vi "VI Server_TextRing_Update_ItemNames.vi"(7 "Label":string, 8 "error in":errorcluster, 10 "Strings []":string[](array[string]), 11 "VI Server Cluster":T1) -> (0 "error out":errorcluster, 1 "Control Reference":refnum<vi>, 3 "VI Server Cluster.DUP":T1)   [LabVIEW 2020, in "VI Server Toolkit LV2013.lvlib"]
doc: "Updates Text Ring Items List."
uses:
  VI Server Toolkit LV2013.lvlib
  VI Server_TypeDefs/VI Server_RefsCluster.ctl
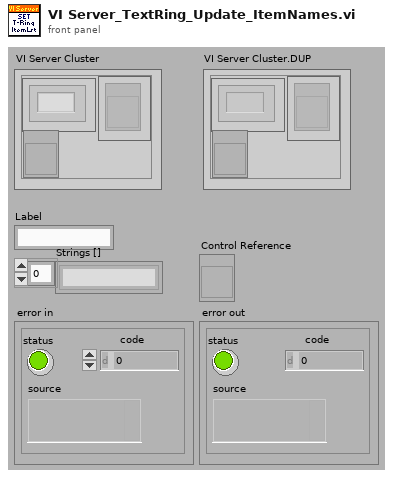
[diagram p1: front panel]
types:
  T1 = typedef "VI Server_RefsCluster.ctl" = cluster{"Labels":string[], "Refs":refnum<vi>[], "VI Ref":refnum<vi>}
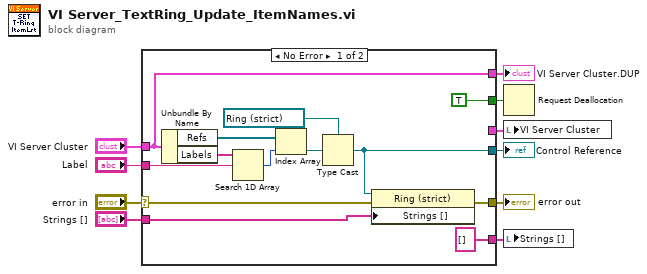
[diagram p0: block diagram]
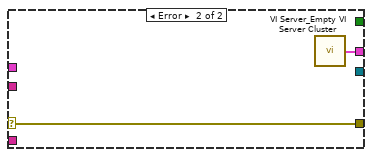
[diagram p2: hidden frame]
diagram:
  n1 = case shown="No Error" "error in" {
    selector: "error in" -> [w17 w25]
    tunnel: "Label" -> [w22 _]
    tunnel: "VI Server Cluster" -> [w13 _]
    tunnel: [w16 w25] -> w10
    tunnel: [w15 _] -> w6
    tunnel: "Strings []" -> [w14 _]
    tunnel: [w13 _] -> w4
    tunnel: [_ w24] -> w3
    tunnel: [string[] [] ("Strings []") _] -> w2
    tunnel: [TRUE _] -> w1
    frame No Error {
      n2 = Unbundle By Name(w13) -> ("Refs"=w20:refnum<vi>[], "Labels"=w23:string[])
      n3 = Search 1D Array(1D array=w23, element=w22) -> (index of element=w21:i32)  [unwired: 1 out]
      n4 = Index Array(array=w20, index=w21) -> (element=w19:refnum<vi>)
      n5 = Type Cast(type=refnum<vi> refnum ("Ring"), x=w19) -> (*(type *) &x=w15:refnum<vi>)
      n6 = property class="Ring (strict)"(reference=w15, error in=w17, "Strings []"=w14) -> (error out=w16:errorcluster)  [unwired: 1 out]
    }
    frame Error {
      n7 = call "VI Server_Empty VI Server Cluster.vi"() -> ("VI Server Cluster"=w24:T1)  [unwired: 7 in]
    }
  }
  "error out" <- w10
  "VI Server Cluster.DUP" <- w4
  "Control Reference" <- w6
  n8 = Request Deallocation(w1) -> ()
  n9 = local write "VI Server Cluster"(w3) -> ()
  n10 = local write "Strings []"(w2) -> ()
